vi "ZK三通阀2操作.vi"(7 "是否启用通讯通知":bool, 8 "error in (no error)":errorcluster, 10 "三通阀2操作":u16(ring) items=["打开三通阀", "关闭三通阀"], 11 "Slave ID":T1) -> (0 "error out":errorcluster)   [LabVIEW 2016, in "质控单元V4.lvlib"]
uses:
  <vilib>/Plasmionique/MB Master/MB_Master/MB_Master.lvclass
  <vilib>/Plasmionique/MB Master/MB Master.lvlib
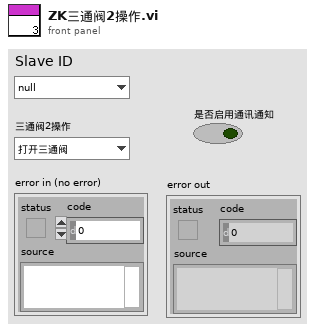
[diagram p1: front panel]
types:
  T1 = typedef "质控单元V4.lvlib/质控slave id.ctl" = enum16{"null", "氨氮", "总磷", "总氮", "CODMn", "CODCr", "氟化物", "挥发酚"}
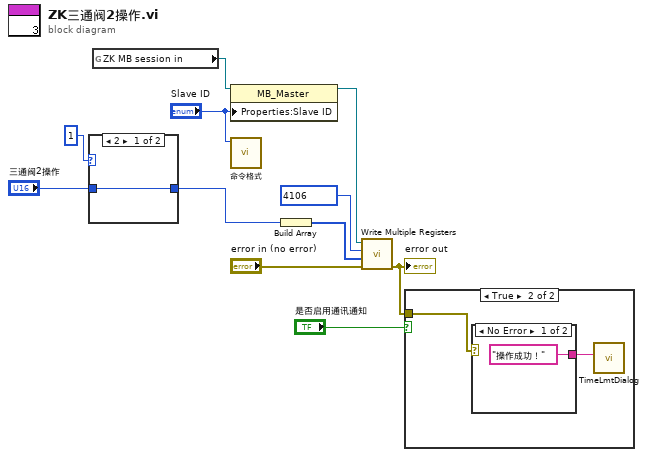
[diagram p0: block diagram]
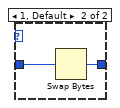
[diagram p2: hidden frame]
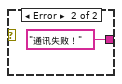
[diagram p4: hidden frame]
diagram:
  n1 = case shown="2" u16 1 ("命令格式") {
    tunnel: "三通阀2操作" -> [w12 w14]
    tunnel: [w12 w13] -> w6
    frame 2 {
    }
    frame 1, Default {
      n2 = Swap Bytes(anything=w14) -> (byte swapped=w13:u16)
    }
  }
  n3 = global read "ZK非断电保存全局变量.vi" "ZK MB session in"() -> (w10:refnum<class "MB_Master.lvclass">)
  n4 = property class="MB_Master"(reference=w10, "Properties:Slave ID"="Slave ID") -> (reference out=w7:refnum<class "MB_Master.lvclass">)  [unwired: 1 in, 1 out]
  n5 = call "命令格式.vi"("站号"="Slave ID") -> ()  [unwired: 10 in, 1 out]
  n6 = Build Array(w6) -> (w5:u16[])
  n7 = call <vilib>:"Write Multiple Registers.vi"("error in (no error)"="error in (no error)", "values"=w5, "starting address"=u16 4106, "MB session in"=w7) -> ("error out"=w4:errorcluster)  [unwired: 6 in, 1 out]
  "error out" <- w4
  n8 = case shown="True" "是否启用通讯通知" {
    tunnel: w4 -> [_ w16]
    frame False {
    }
    frame True {
      n9 = case shown="No Error" w16 {
        tunnel: ["操作成功！" "通讯失败！"] -> w15
        frame No Error {
        }
        frame Error {
        }
      }
      n10 = call "TimeLmtDialog.vi"("Infoin"=w15) -> ()  [unwired: 11 in]
    }
  }
